vi "DeleteLayer.vi"(6 "error in":errorcluster, 7 "AntsRect":T8, 9 "Data in":T1={"Class"={"Ants"=refnum, "Layer"=refnum, "Templates"=refnum, "Icon"=refnum, "Glyph"=refnum, "Settings"=refnum, "Tools"=refnum}, "Ref"={"Add Layer"=refnum, "Remove Layer"=refnum, "Line Text"=[], "Body Text Spec"=refnum, "DNL_Font"=refnum, "glyph path str"=refnum, "templates path str"=refnum, "Arrow Up"=refnum, "Arrow Down"=refnum, "IE VI Ref"=refnum, "Glyphs tree"=refnum, "Templates tree"=refnum, "Layer Icon Text"=refnum, "Layer Template"=refnum, "Body Text"=refnum, "Search Templates"=refnum, "TextMarker"=refnum, "Tab Control"=refnum, "Search Glyphs"=refnum, "Line Color"=refnum, "DNL_Glyphs []"=refnum, "Fill Color"=refnum, "Tools"=refnum, "Icon"=refnum, "Preview"=refnum, "Ants"=refnum, "Terminals"=refnum, "menu reference"=refnum, "LayerNames"=[], "GlyphLoadAnimation"=refnum, "TemplateLoadAnimation"=refnum, "refreshGlyphs"=refnum, "refreshTemplates"=refnum}, "Support"={"AntsRect"={"left"=0, "top"=0, "right"=0, "bottom"=0}, "Mouse Move Coords"={"Horizontal"=0, "Vertical"=0}, "Mouse Down Coords"={"Horizontal"=0, "Vertical"=0}, "Temp Coord"={"Horizontal"=0, "Vertical"=0}, "Action"=enum."Default", "Edge Color"=4914962, "Fill Color"=16860, "Mouse Down?"=FALSE, "Draft Mode?"=FALSE, "Temp Icon"=bytes[3102], "CTRL Pressed"=FALSE, "Move Selection?"=FALSE, "AntsRect Orig"={"left"=0, "top"=0, "right"=0, "bottom"=0}, "Text"="", "TM Set?"=FALSE, "Mouse inside icon?"=FALSE, "Tool (old value)"=0, "Pencil Move Color"=0, "Swap Colors?"=FALSE, "Shift pressed?"=FALSE}}) -> (0 "error out":errorcluster, 3 "Data out":T1={"Class"={"Ants"=refnum, "Layer"=refnum, "Templates"=refnum, "Icon"=refnum, "Glyph"=refnum, "Settings"=refnum, "Tools"=refnum}, "Ref"={"Add Layer"=refnum, "Remove Layer"=refnum, "Line Text"=[], "Body Text Spec"=refnum, "DNL_Font"=refnum, "glyph path str"=refnum, "templates path str"=refnum, "Arrow Up"=refnum, "Arrow Down"=refnum, "IE VI Ref"=refnum, "Glyphs tree"=refnum, "Templates tree"=refnum, "Layer Icon Text"=refnum, "Layer Template"=refnum, "Body Text"=refnum, "Search Templates"=refnum, "TextMarker"=refnum, "Tab Control"=refnum, "Search Glyphs"=refnum, "Line Color"=refnum, "DNL_Glyphs []"=refnum, "Fill Color"=refnum, "Tools"=refnum, "Icon"=refnum, "Preview"=refnum, "Ants"=refnum, "Terminals"=refnum, "menu reference"=refnum, "LayerNames"=[], "GlyphLoadAnimation"=refnum, "TemplateLoadAnimation"=refnum, "refreshGlyphs"=refnum, "refreshTemplates"=refnum}, "Support"={"AntsRect"={"left"=0, "top"=0, "right"=0, "bottom"=0}, "Mouse Move Coords"={"Horizontal"=0, "Vertical"=0}, "Mouse Down Coords"={"Horizontal"=0, "Vertical"=0}, "Temp Coord"={"Horizontal"=0, "Vertical"=0}, "Action"=enum."Default", "Edge Color"=4914962, "Fill Color"=16860, "Mouse Down?"=FALSE, "Draft Mode?"=FALSE, "Temp Icon"=bytes[3102], "CTRL Pressed"=FALSE, "Move Selection?"=FALSE, "AntsRect Orig"={"left"=0, "top"=0, "right"=0, "bottom"=0}, "Text"="", "TM Set?"=FALSE, "Mouse inside icon?"=FALSE, "Tool (old value)"=0, "Pencil Move Color"=0, "Swap Colors?"=FALSE, "Shift pressed?"=FALSE}})   [LabVIEW 2021]
uses:
  <resource>/plugins/NIIconEditor/Controls/Global Data.ctl
  <resource>/plugins/NIIconEditor/Class/Ants/Ants.lvclass
  <resource>/plugins/NIIconEditor/Class/FakedArray/FakedArray.lvclass
  <vilib>/LabVIEW Icon API/lv_icon/Classes/Icon/Icon.lvclass
  <resource>/plugins/NIIconEditor/Class/Icon Library/Glyph.lvclass
  <resource>/plugins/NIIconEditor/Class/Settings/Settings.lvclass
  <resource>/plugins/NIIconEditor/Class/Tools/Tools Paint.lvclass
  <resource>/plugins/NIIconEditor/Controls/IE Classes.ctl
  <resource>/plugins/NIIconEditor/Controls/References Cluster.ctl
  <resource>/plugins/NIIconEditor/Controls/SupportClass.ctl
  <vilib>/Utility/miscctls.llb/LVPoint32TypeDef.ctl
  <resource>/plugins/NIIconEditor/Controls/SupportClass_Action.ctl
  <vilib>/LabVIEW Icon API/lv_icon/Controls/IEColor.ctl
  <vilib>/LabVIEW Icon API/lv_icon/Classes/Layer/Layer.lvclass
  <vilib>/LabVIEW Icon API/lv_icon/lv_icon.lvlib
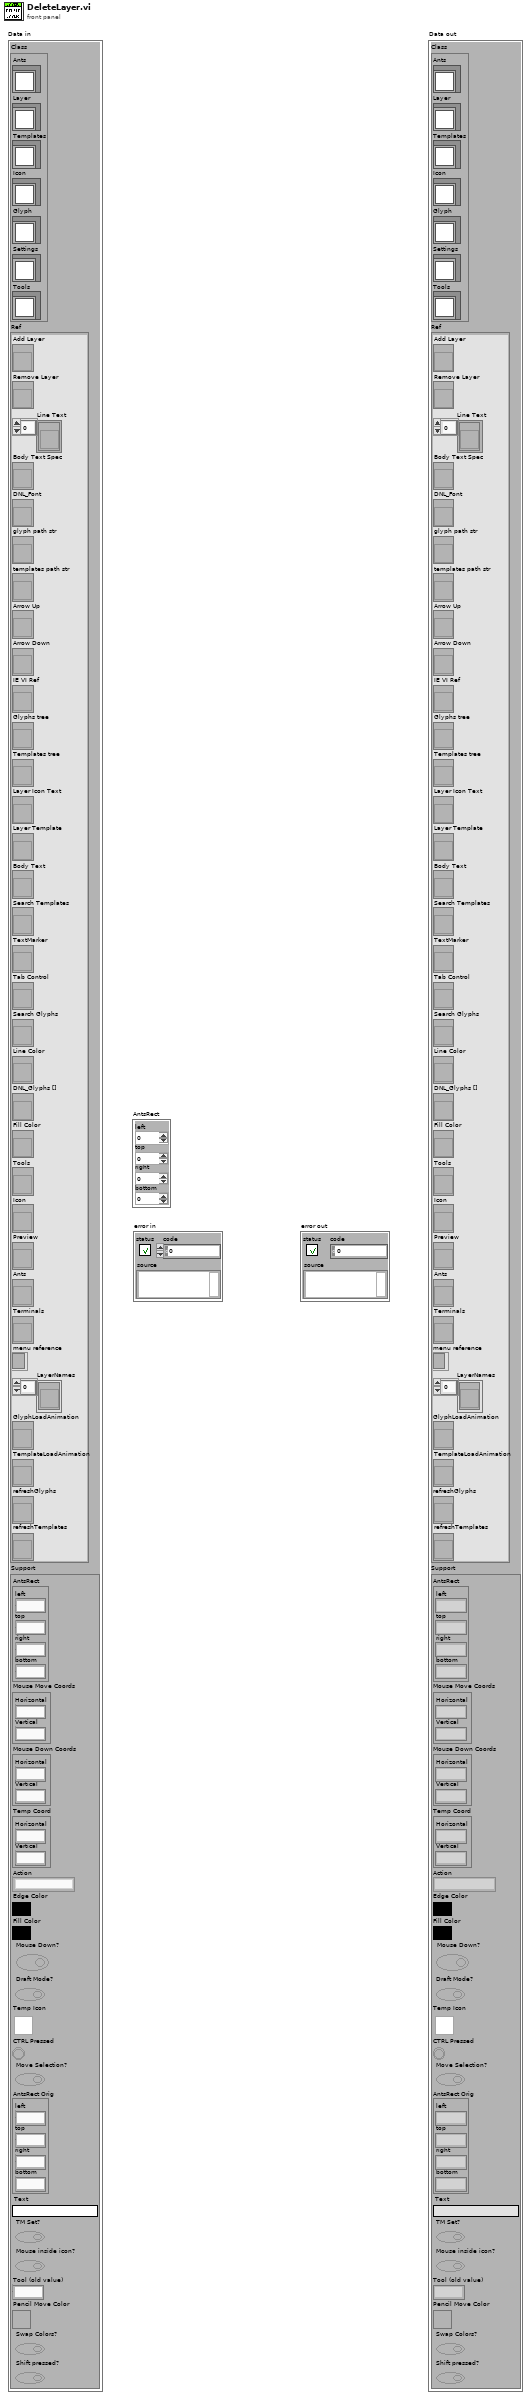
[diagram p1: front panel]
types:
  T1 = typedef "lv_icon.lvlib/Global Data.ctl" = cluster{"Class":T2, "Ref":T3, "Support":T4}
  T2 = typedef "IE Classes.ctl" = cluster{"Ants":refnum<class "Ants.lvclass">, "Layer":refnum<class "FakedArray.lvclass">, "Templates":refnum<class "FakedArray.lvclass">, "Icon":refnum<class "Icon.lvclass">, "Glyph":refnum<class "Glyph.lvclass">, "Settings":refnum<class "Settings.lvclass">, "Tools":refnum<class "Tools Paint.lvclass">}
  T3 = typedef "lv_icon.lvlib/References Cluster.ctl" = cluster{"Add Layer":refnum<vi>, "Remove Layer":refnum<vi>, "Line Text":refnum<vi>[], "Body Text Spec":refnum<vi>, "DNL_Font":refnum<vi>, "glyph path str":refnum<vi>, "templates path str":refnum<vi>, "Arrow Up":refnum<vi>, "Arrow Down":refnum<vi>, "IE VI Ref":refnum<vi>, "Glyphs tree":refnum<vi>, "Templates tree":refnum<vi>, "Layer Icon Text":refnum<vi>, "Layer Template":refnum<vi>, "Body Text":refnum<vi>, "Search Templates":refnum<vi>, "TextMarker":refnum<vi>, "Tab Control":refnum<vi>, "Search Glyphs":refnum<vi>, "Line Color":refnum<vi>, "DNL_Glyphs []":refnum<vi>, "Fill Color":refnum<vi>, "Tools":refnum<vi>, "Icon":refnum<vi>, "Preview":refnum<vi>, "Ants":refnum<vi>, "Terminals":refnum<vi>, "menu reference":refnum<k9>, "LayerNames":refnum<vi>[], "GlyphLoadAnimation":refnum<vi>, "TemplateLoadAnimation":refnum<vi>, "refreshGlyphs":refnum<vi>, "refreshTemplates":refnum<vi>}
  T4 = typedef "SupportClass.ctl" = cluster{"AntsRect":cluster{"left":i16, "top":i16, "right":i16, "bottom":i16}, "Mouse Move Coords":T5, "Mouse Down Coords":T5, "Temp Coord":T5, "Action":T6, "Edge Color":T7, "Fill Color":T7, "Mouse Down?":bool, "Draft Mode?":bool, "Temp Icon":picture, "CTRL Pressed":bool, "Move Selection?":bool, "AntsRect Orig":cluster{"left":i16, "top":i16, "right":i16, "bottom":i16}, "Text":string, "TM Set?":bool, "Mouse inside icon?":bool, "Tool (old value)":u32, "Pencil Move Color":u32, "Swap Colors?":bool, "Shift pressed?":bool}
  T5 = typedef "LVPoint32TypeDef.ctl" = cluster{"Horizontal":i32, "Vertical":i32}
  T6 = typedef "SupportClass_Action.ctl" = enum16{"Default", "Move Selection", "Glyph Library", "Tool"}
  T7 = typedef "IEColor.ctl" = u32
  T8 = cluster{"left":i16, "top":i16, "right":i16, "bottom":i16}
  T9 = typedef "Layer.ctl" = cluster{"LayerIcon":picture, "LayerName":string, "Opacity":u8, "Visibility?":bool}
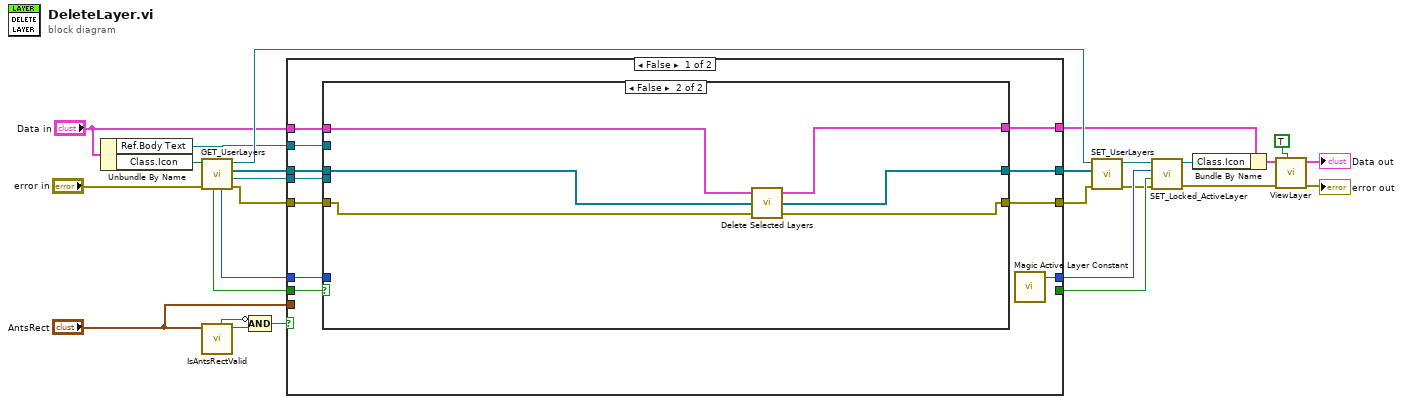
[diagram p0: block diagram]
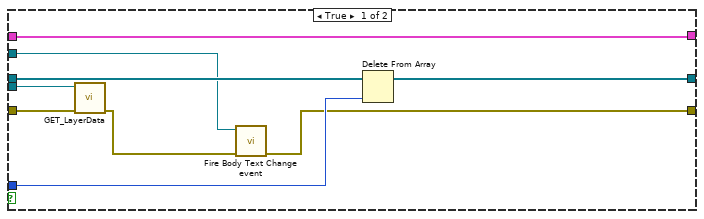
[diagram p2: hidden frame]
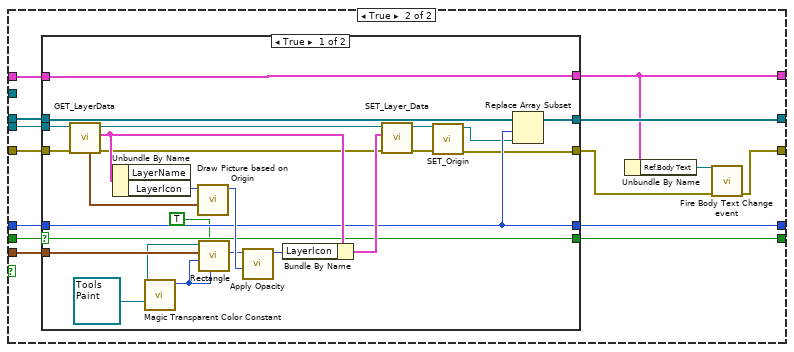
[diagram p3: hidden frame]
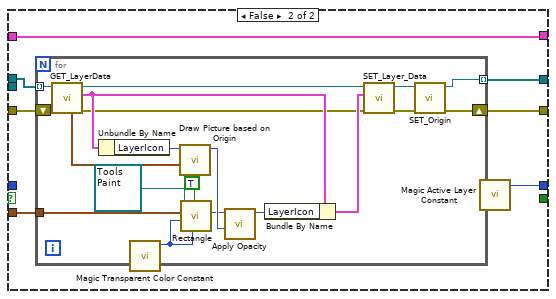
[diagram p4: hidden frame]
diagram:
  n1 = Unbundle By Name("Data in") -> ("Ref.Body Text"=w1:refnum<vi>, "Class.Icon"=w16:refnum<class "Icon.lvclass">)
  n2 = call-dynamic "GET_UserLayers.vi"("error in (no error)"="error in", "Icon.lvclass in"=w16) -> ("error out"=w24:errorcluster, "Active Layer"=w22:refnum<class "Layer.lvclass">, "All Layers"=w23:refnum<class "Layer.lvclass">[], "Icon.lvclass out"=w26:refnum<class "Icon.lvclass">, "#Active Layer"=w25:i32, "Layer Locked?"=w21:bool)  [unwired: 4 out]
  n3 = call <resource>:"IsAntsRectValid.vi"("AntsRect"="AntsRect") -> ("Valid?"=w4:bool, "Max. Rect size?"=w3:bool)  [unwired: 9 out]
  n4 = Compound Arithmetic op=AND(invert w3, w4) -> (w2:bool)
  n5 = case shown="False" w2 {
    tunnel: [w38 w56] -> w27
    tunnel: [w37 w61] -> w5
    tunnel: w25 -> [w36 w66]
    tunnel: w24 -> [w35 w64]
    tunnel: w23 -> [w34 w62]
    tunnel: w22 -> [w33 w65]
    tunnel: w21 -> [w32 w67]
    tunnel: "AntsRect" -> [_ w63]
    tunnel: [w31 w60] -> w19
    tunnel: [_ w59] -> w18
    tunnel: "Data in" -> [w30 w58]
    tunnel: [w29 w55] -> w13
    tunnel: w1 -> [w28 _]
    frame False {
      n6 = case shown="False" w32 {
        tunnel: w33 -> [w44 _]
        tunnel: w34 -> [w47 w53]
        tunnel: w35 -> [w43 w49]
        tunnel: w36 -> [w45 _]
        tunnel: [w46 w52] -> w37
        tunnel: [w41 w51] -> w38
        tunnel: w30 -> [w40 w50]
        tunnel: [w40 w48] -> w29
        tunnel: w28 -> [w39 _]
        frame True {
          n7 = call-dynamic "GET_LayerData.vi"("error in (no error)"=w43, "Layer.lvclass in"=w44) -> ("error out"=w42:errorcluster)  [unwired: 9 out]
          n8 = call <resource>:"Fire Body Text Change event.vi"("error in"=w42, "Ref.Body Text"=w39) -> ("error out"=w41:errorcluster)  [unwired: 2 in, 7 out]
          n9 = Delete From Array(array=w47, index=w45) -> (array with subset deleted=w46:refnum<class "Layer.lvclass">[])  [unwired: 1 in, 1 out]
        }
        frame False {
          n10 = call <resource>:"Delete Selected Layers.vi"("error in"=w49, "All Layers in"=w53, "Data in"=w50) -> ("error out"=w51:errorcluster, "All Layers out"=w52:refnum<class "Layer.lvclass">[], "Data out"=w48:T1)
        }
      }
      n11 = call <resource>:"Magic Active Layer Constant.vi"() -> ("Magic Constant"=w31:i32)  [unwired: 19 out]
    }
    frame True {
      n12 = case shown="True" w67 {
        selector: w67 -> [w77 _]
        tunnel: w66 -> [w78 _]
        tunnel: w65 -> [w91 _]
        tunnel: w64 -> [w90 w98]
        tunnel: w63 -> [w87 w97]
        tunnel: [w70 w96] -> w57
        tunnel: w62 -> [w80 w95]
        tunnel: [w79 w94] -> w61
        tunnel: [w78 w93] -> w60
        tunnel: [w77 _] -> w59
        tunnel: w58 -> [w69 w92]
        tunnel: [w69 w92] -> w55
        frame True {
          n13 = call-dynamic "GET_LayerData.vi"("error in (no error)"=w90, "Layer.lvclass in"=w91) -> ("error out"=w68:errorcluster, "Data"=w84:T9, "Layer.lvclass out"=w82:refnum<class "Layer.lvclass">, "Origin"=w88:T5)  [unwired: 6 out]
          n14 = Unbundle By Name(w84) -> ("LayerIcon"=w89:picture)  [unwired: 1 out]
          n15 = call <vilib>:"Magic Transparent Color Constant.vi"() -> ("Magic transparent color constant"=w74:u32)  [unwired: 11 out]
          n16 = call <vilib>:"Draw Picture based on Origin.vi"("Origin"=w88, "LayerIcon in"=w89) -> ("LayerIcon out"=w86:picture)  [unwired: 1 in, 8 out]
          n17 = call-dynamic "Rectangle.vi"("Fill Color"=w74, "fill?(F)"=TRUE, "Edge Color"=w74, "rect"=w87, "Tools Paint in"=refnum<class "Tools Paint.lvclass"> refnum) -> ("new picture"=w85:picture)  [unwired: 1 in, 5 out]
          n18 = call <vilib>:"Apply Opacity.vi"("Bottom"=w86, "Top"=w85) -> ("new picture"=w83:picture)  [unwired: 1 in, 8 out]
          n19 = Bundle By Name(cluster=w84, "LayerIcon"=w83) -> (w81:T9)
          n20 = call-dynamic "SET_Layer_Data.vi"("error in (no error)"=w68, "Data"=w81, "Layer.lvclass in"=w82) -> ("error out"=w72:errorcluster, "Layer.lvclass out"=w73:refnum<class "Layer.lvclass">)  [unwired: 1 in, 6 out]
          n21 = call-dynamic "SET_Origin.vi"("error in (no error)"=w72, "Layer.lvclass in"=w73) -> ("error out"=w70:errorcluster, "Layer.lvclass out"=w71:refnum<class "Layer.lvclass">)  [unwired: 8 in]
          n22 = Replace Array Subset(array=w80, new element=w71, index=w78) -> (w79:refnum<class "Layer.lvclass">[])
        }
        frame False {
          n23 = for {
            tunnel: w97 -> [w114]
            shift-right: [w100] -> w96
            shift-left: w98 -> [w117]
            tunnel: w95 -> [w107] mode=indexing
            tunnel: [w101] -> w94 mode=indexing
            n24 = call-dynamic "GET_LayerData.vi"("error in (no error)"=w117, "Layer.lvclass in"=w107) -> ("error out"=w99:errorcluster, "Data"=w111:T9, "Layer.lvclass out"=w109:refnum<class "Layer.lvclass">, "Origin"=w115:T5)  [unwired: 6 out]
            n25 = Unbundle By Name(w111) -> ("LayerIcon"=w116:picture)
            n26 = call <vilib>:"Magic Transparent Color Constant.vi"() -> ("Magic transparent color constant"=w104:u32)  [unwired: 11 out]
            n27 = call <vilib>:"Draw Picture based on Origin.vi"("Origin"=w115, "LayerIcon in"=w116) -> ("LayerIcon out"=w113:picture)  [unwired: 1 in, 8 out]
            n28 = call-dynamic "Rectangle.vi"("Fill Color"=w104, "fill?(F)"=TRUE, "Edge Color"=w104, "rect"=w114, "Tools Paint in"=refnum<class "Tools Paint.lvclass"> refnum) -> ("new picture"=w112:picture)  [unwired: 1 in, 5 out]
            n29 = call <vilib>:"Apply Opacity.vi"("Bottom"=w113, "Top"=w112) -> ("new picture"=w110:picture)  [unwired: 1 in, 8 out]
            n30 = Bundle By Name(cluster=w111, "LayerIcon"=w110) -> (w108:T9)
            n31 = call-dynamic "SET_Layer_Data.vi"("error in (no error)"=w99, "Data"=w108, "Layer.lvclass in"=w109) -> ("error out"=w103:errorcluster, "Layer.lvclass out"=w102:refnum<class "Layer.lvclass">)  [unwired: 1 in, 6 out]
            n32 = call-dynamic "SET_Origin.vi"("error in (no error)"=w103, "Layer.lvclass in"=w102) -> ("error out"=w100:errorcluster, "Layer.lvclass out"=w101:refnum<class "Layer.lvclass">)  [unwired: 8 in]
          }
          n33 = call <resource>:"Magic Active Layer Constant.vi"() -> ("Magic Constant"=w93:i32)  [unwired: 19 out]
        }
      }
      n34 = Unbundle By Name(w55) -> ("Ref.Body Text"=w54:refnum<vi>)
      n35 = call <resource>:"Fire Body Text Change event.vi"("error in"=w57, "Ref.Body Text"=w54) -> ("error out"=w56:errorcluster)  [unwired: 2 in, 7 out]
    }
  }
  n36 = call-dynamic "SET_UserLayers.vi"("error in (no error)"=w27, "Layers"=w5, "Icon.lvclass in"=w26) -> ("error out"=w11:errorcluster, "Icon.lvclass out"=w10:refnum<class "Icon.lvclass">)  [unwired: 7 in]
  n37 = call-dynamic "SET_Locked_ActiveLayer.vi"("error in (no error)"=w11, "Layers Locked?"=w18, "Active Layer"=w19, "Icon.lvclass in"=w10) -> ("error out"=w6:errorcluster, "Icon.lvclass out"=w14:refnum<class "Icon.lvclass">)  [unwired: 6 out]
  n38 = Bundle By Name(cluster=w13, "Class.Icon"=w14) -> (w9:T1)
  n39 = call <resource>:"ViewLayer.vi"("Add to Undo?"=TRUE, "error in (no error)"=w6, "Data in"=w9) -> ("error out"=→"error out":errorcluster, "Data out"=→"Data out":T1)  [unwired: 1 in, 6 out]
